vi "Power Availability Requests.vi"(8 "error in (no error)":errorcluster, 9 "Simple Reason String":string, 10 "Power Request Type":T1, 11 "Power Availability Requests Functions":T2) -> (0 "error out":errorcluster, 3 "Success?":bool)   [LabVIEW 2016, in "Power Requests.lvlib"]
uses:
  <userlib>/Power-Requests-master/Power Requests.lvlib
  <userlib>/Power-Requests-master/Power Availabilty Requests/Type Defs/Power Availiability Requests Functions.ctl
  <userlib>/Power-Requests-master/Power Availabilty Requests/Type Defs/Power Request Type.ctl
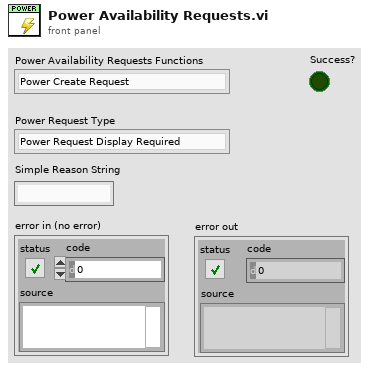
[diagram p1: front panel]
types:
  T1 = typedef "Power Requests.lvlib/Power Request Type.ctl" = enum32{"Power Request Display Required", "Power Request System Required", "Power Request Away Mode Required", "Power Request Execution Required"}
  T2 = typedef "Power Requests.lvlib/Power Availiability Requests Functions.ctl" = enum32{"Power Create Request", "Power Set Request", "Power Clear Request", "Close Handle"}
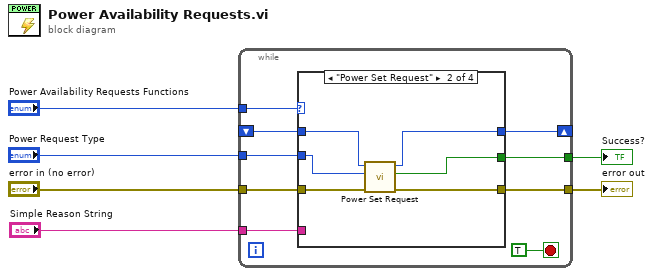
[diagram p0: block diagram]
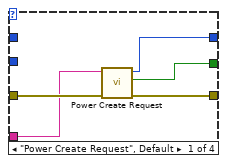
[diagram p2: hidden frame]
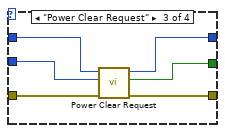
[diagram p3: hidden frame]
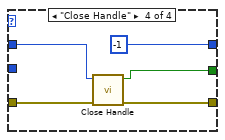
[diagram p4: hidden frame]
diagram:
  n1 = while {
    shift-right: [w10] -> _
    shift-left: _ -> [w8]
    tunnel: "Power Availability Requests Functions" -> [w14]
    tunnel: "error in (no error)" -> [w13]
    tunnel: "Power Request Type" -> [w12]
    tunnel: [w11] -> w2
    tunnel: "Simple Reason String" -> [w9]
    tunnel: [w7] -> w1
    stop <- TRUE stop-if-true
    n2 = case shown="\"Power Set Request\"" w14 {
      tunnel: w13 -> [w20 w26 w32 w37]
      tunnel: w12 -> [_ w22 w28 _]
      tunnel: [w19 w25 w31 w36] -> w11
      tunnel: [w18 w23 w29 i64 -1 ("Handle out")] -> w10
      tunnel: w9 -> [w17 _ _ _]
      tunnel: w8 -> [_ w24 w30 w35]
      tunnel: [w16 w21 w27 w33] -> w7
      frame "Power Create Request", Default {
        n3 = call <userlib>:"Power Create Request.vi"("error in (no error)"=w20, "Simple Reason String"=w17) -> ("error out"=w19:errorcluster, "Success?"=w16:bool, "Handle"=w18:i64)  [unwired: 7 in]
      }
      frame "Power Set Request" {
        n4 = call <userlib>:"Power Set Request.vi"("error in (no error)"=w26, "Power Request Type"=w22, "Handle in"=w24) -> ("error out"=w25:errorcluster, "Success?"=w21:bool, "Handle out"=w23:i64)  [unwired: 6 in]
      }
      frame "Power Clear Request" {
        n5 = call <userlib>:"Power Clear Request.vi"("error in (no error)"=w32, "Power Request Type"=w28, "Handle in"=w30) -> ("error out"=w31:errorcluster, "Success?"=w27:bool, "Handle out"=w29:i64)  [unwired: 6 in]
      }
      frame "Close Handle" {
        n6 = call <userlib>:"Close Handle.vi"("error in (no error)"=w37, "Handle"=w35) -> ("error out"=w36:errorcluster, "Sucess?"=w33:bool)  [unwired: 8 in]
      }
    }
  }
  "error out" <- w2
  "Success?" <- w1
